vi "CircularRadius.vi"(5 "Direction":u16(ring) items=["Clockwise", "Counter-clockwise"], 6 "radius":dbl, 8 "Speed":dbl, 9 "XY End":dbl[](array[numeric]), 11 "Gantry in":refnum<class "A3200.lvclass">) -> (3 "Gantry out":refnum<class "A3200.lvclass">)   [LabVIEW 2016, in "A3200.lvclass"]
uses:
  A3200.lvclass
  A3200.lvclass/A3200.ctl
  <userlib>/Aerotech A3200.lnk/Aerotech VIs.lvlib
panel:
  out "error out":errorcluster
  in  "error in (no error)":errorcluster
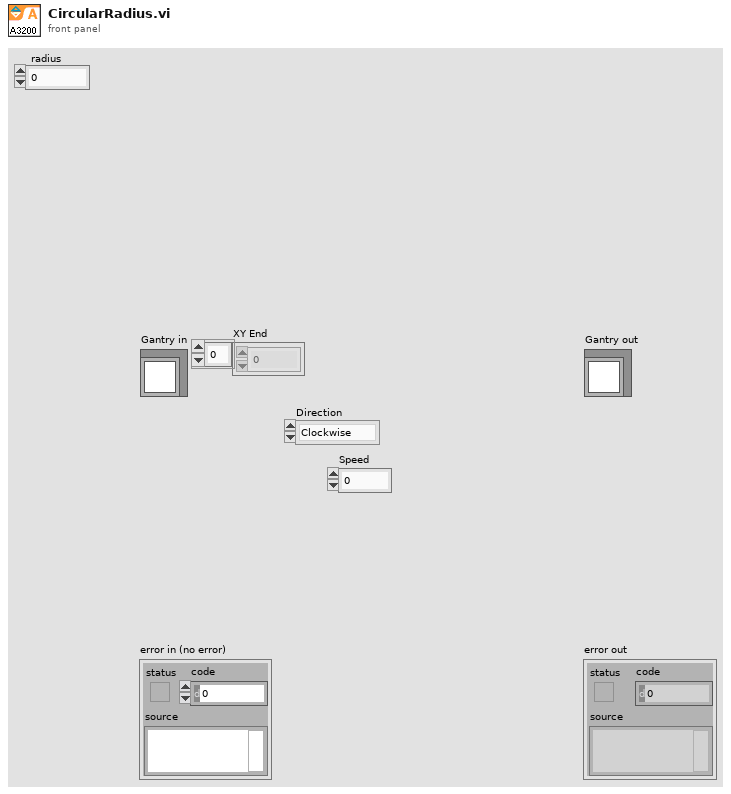
[diagram p1: front panel]
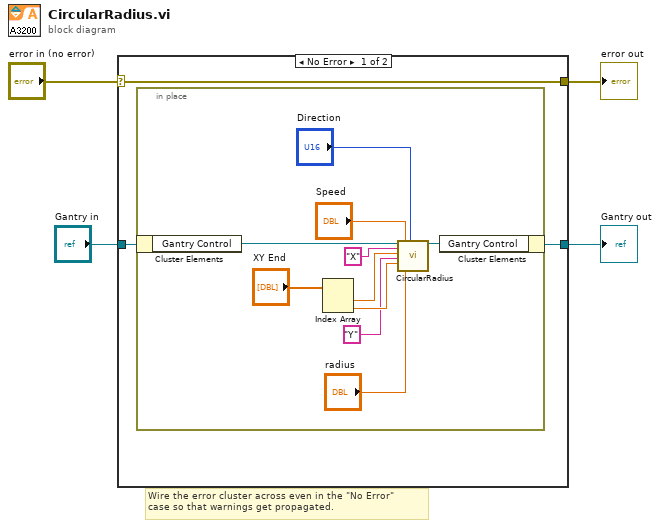
[diagram p0: block diagram]
diagram:
  # "Wire the error cluster across even in the \"No Error\"\ncase so that warnings get propagated."
  n1 = case shown="No Error" "error in (no error)" {
    selector: "error in (no error)" -> [w7 w19]
    tunnel: [w7 w19] -> w3
    tunnel: [w5 w18] -> w1
    tunnel: "Gantry in" -> [w6 w18]
    frame No Error {
      n2 = in-place {
        n3 = in-place-cluster #1(w6) -> ("Gantry Control"=w9:refnum<k24>)
        n4 = Index Array(array="XY End") -> (element #1=w15:dbl, element #2=w14:dbl)  [unwired: 2 in]
        n5 = call <userlib>:"CircularRadius.vi"("controller in"=w9, "axis 1 name"="X", "axis 1 endpoint"=w15, "axis 2 name"="Y" ("axis 1 name"), "axis 2 endpoint"=w14, "speed"="Speed", "radius"="radius", "direction"="Direction") -> ("controller out"=w8:refnum<k24>)  [unwired: 10 in, 1 out]
        n6 = in-place-cluster #1("Gantry Control"=w8) -> (w5:refnum<class "A3200.lvclass">)
      }
    }
    frame Error {
    }
  }
  "error out" <- w3
  "Gantry out" <- w1
